vi "Facade 3.vi"(0 "Data In":T4, 2 "Display State In":T2, 3 "Container State":T3) -> (6 "Data Out":T4, 7 "Display State Out":T2, 8 "Action":T1)   [LabVIEW 2021, in "溫度計.xctl"]
uses:
  Data 3.ctl
  <vilib>/_xctls/Container State.ctl
  State 3.ctl
  <vilib>/_xctls/Action.ctl
  <vilib>/_xctls/XControlSupport.lvlib
panel:
  in  "下限":dbl
  in  "圖片異常":path
  in  "圖片正常":path
  out "訊息":string
  in  "上限":dbl
  out "顯示圖片":picture
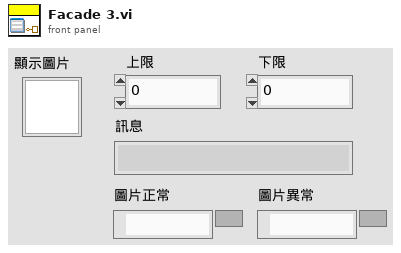
[diagram p1: front panel]
types:
  T1 = typedef "XControlSupport.lvlib/Action.ctl" = cluster{"Data Changed?":bool, "State Changed?":bool, "Action Name":string}
  T2 = typedef "溫度計.xctl/State 3.ctl" = cluster{"Numeric":dbl}
  T3 = typedef "XControlSupport.lvlib/Container State.ctl" = cluster{"Indicator?":bool, "Run Mode?":bool, " Refnum":refnum<vi>}
  T4 = typedef "溫度計.xctl/Data 3.ctl" = dbl
  T5 = typedef "imagedata.ctl" = cluster{"image type":i32, "image depth":i32, "image":u8[], "mask":u8[], "colors":u32[], "Rectangle":cluster{"left":i16, "top":i16, "right":i16, "bottom":i16}}
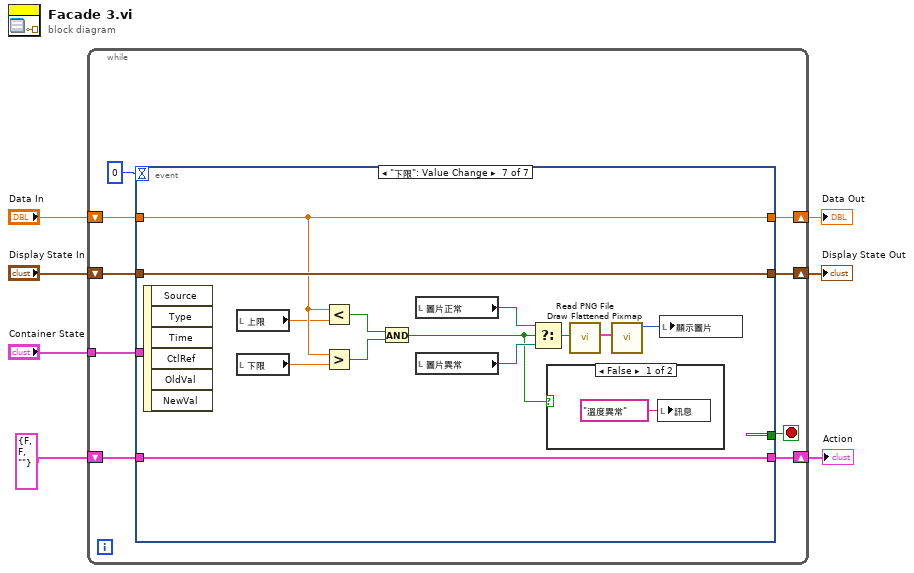
[diagram p0: block diagram]
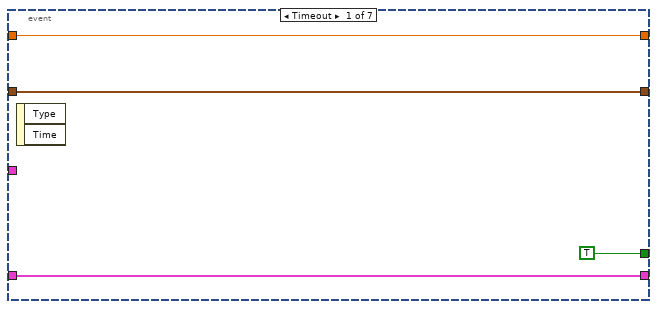
[diagram p2: hidden frame]
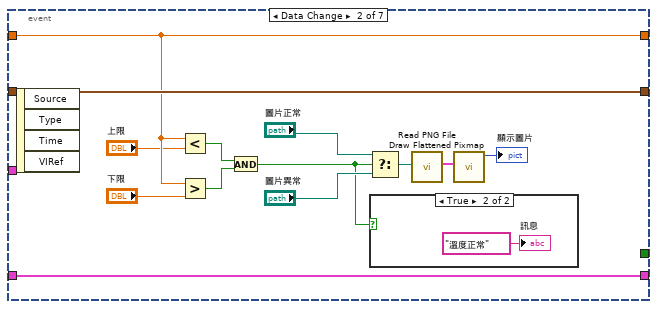
[diagram p3: hidden frame]
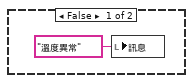
[diagram p4: hidden frame]
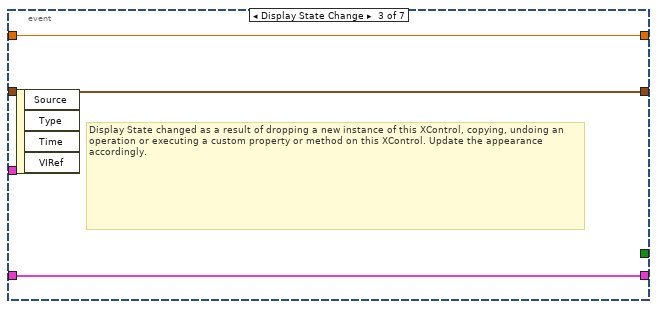
[diagram p5: hidden frame]
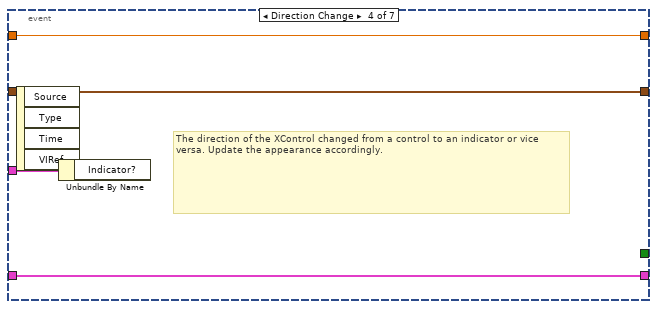
[diagram p6: hidden frame]
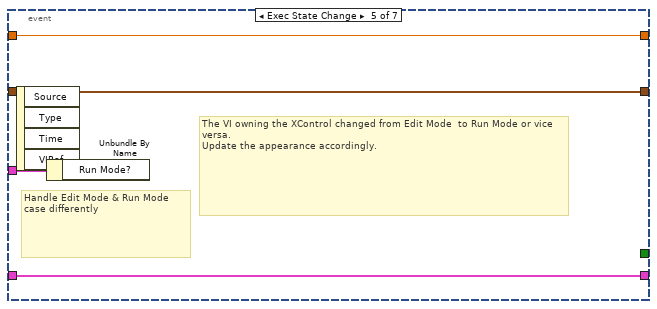
[diagram p7: hidden frame]
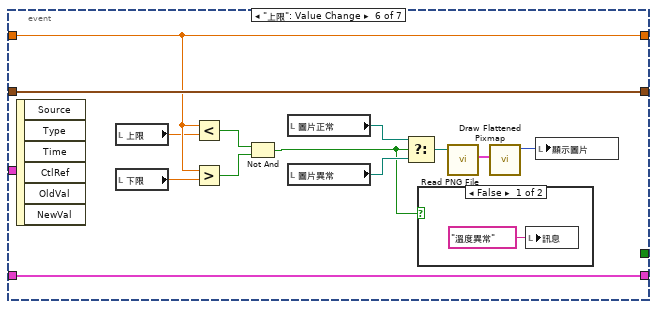
[diagram p8: hidden frame]
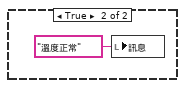
[diagram p9: hidden frame]
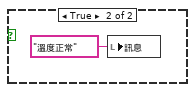
[diagram p10: hidden frame]
diagram:
  n1 = while {
    shift-right: [w15] -> w4
    shift-left: "Display State In" -> [w16]
    tunnel: "Container State" -> [w12]
    shift-right: [w10] -> w7
    shift-left: "Data In" -> [w11]
    shift-right: [w8] -> w2
    shift-left: T1 {"Data Changed?"=FALSE, "State Changed?"=FALSE, "Action Name"=""} ("Action") -> [w9]
    stop <- w14 stop-if-true
    n2 = event shown="[6] \"下限\": Value Change" {
      selector: _ -> [_ _ _ _ _ _ _]
      dyn-events: _ -> [_ _ _ _ _ _ _]
      timeout: 0 -> [_ _ _ _ _ _ _]
      tunnel: w16 -> [w18 w33 w38 w41 w45 w59 w74]
      tunnel: [w18 w33 w38 w41 w45 w59 w74] -> w15
      tunnel: [TRUE _ _ _ _ _ _] -> w14
      tunnel: w12 -> [_ _ _ w42 w46 _ _]
      tunnel: w11 -> [w17 w26 w37 w40 w44 w52 w67]
      tunnel: [w17 w26 w37 w40 w44 w52 w67] -> w10
      tunnel: [w19 w32 w36 w39 w43 w58 w73] -> w8
      tunnel: w9 -> [w19 w32 w36 w39 w43 w58 w73]
      event Timeout {
        n3 = event-data() -> ()  [unwired: 1 in, 2 out]
      }
      event Data Change {
        n4 = event-data() -> ()  [unwired: 1 in, 4 out]
        n5 = Less?(x=w26, y="上限") -> (x < y?=w23:bool)
        n6 = Greater?(x=w26, y="下限") -> (0:w22:bool)
        n7 = And(x=w23, y=w22) -> (x .and. y?=w21:bool)
        n8 = Select(t="圖片正常", s=w21, f="圖片異常") -> (s? t:f=w30:path)
        n9 = case shown="True" w21 {
          frame False {
            n10 = local write "訊息"("溫度異常" ("訊息")) -> ()
          }
          frame True {
            "訊息" <- "溫度正常" ("訊息")
          }
        }
        n11 = call <vilib>:"Read PNG File.vi"("path to PNG file"=w30) -> ("image data"=w27:T5)  [unwired: 8 in, 2 out]
        n12 = call <vilib>:"Draw Flattened Pixmap.vi"("image data"=w27) -> ("new picture"=→"顯示圖片":picture)  [unwired: 8 in]
      }
      event Display State Change {
        # "Display State changed as a result of dropping a new instance of this XControl, copying, undoing an operation or executing a custom property or method on this XControl. Update the appearance accordingly."
        n13 = event-data() -> ()  [unwired: 1 in, 4 out]
      }
      event Direction Change {
        # "The direction of the XControl changed from a control to an indicator or vice versa. Update the appearance accordingly."
        n14 = event-data() -> ()  [unwired: 1 in, 4 out]
        n15 = Unbundle By Name(w42) -> ()  [unwired: 1 out]
      }
      event Exec State Change {
        # "The VI owning the XControl changed from Edit Mode  to Run Mode or vice versa.\nUpdate the appearance accordingly."
        # "Handle Edit Mode & Run Mode\ncase differently"
        n16 = event-data() -> ()  [unwired: 1 in, 4 out]
        n17 = Unbundle By Name(w46) -> ()  [unwired: 1 out]
      }
      event "上限": Value Change {
        n18 = event-data() -> ()  [unwired: 1 in, 6 out]
        n19 = local read "上限"() -> (w51:dbl)
        n20 = local read "下限"() -> (w50:dbl)
        n21 = Less?(x=w52, y=w51) -> (x < y?=w49:bool)
        n22 = Greater?(x=w52, y=w50) -> (0:w48:bool)
        n23 = Not And(1:w48, 2:w49) -> (0:w47:bool)
        n24 = local read "圖片正常"() -> (w54:path)
        n25 = local read "圖片異常"() -> (w53:path)
        n26 = Select(t=w54, s=w47, f=w53) -> (s? t:f=w55:path)
        n27 = case shown="False" w47 {
          frame False {
            n28 = local write "訊息"("溫度異常" ("訊息")) -> ()
          }
          frame True {
            n29 = local write "訊息"("溫度正常" ("訊息")) -> ()
          }
        }
        n30 = call <vilib>:"Read PNG File.vi"("path to PNG file"=w55) -> ("image data"=w57:T5)  [unwired: 8 in, 2 out]
        n31 = call <vilib>:"Draw Flattened Pixmap.vi"("image data"=w57) -> ("new picture"=w56:picture)  [unwired: 8 in]
        n32 = local write "顯示圖片"(w56) -> ()
      }
      event "下限": Value Change {
        n33 = event-data() -> ()  [unwired: 1 in, 6 out]
        n34 = local read "上限"() -> (w66:dbl)
        n35 = local read "下限"() -> (w65:dbl)
        n36 = Less?(x=w67, y=w66) -> (x < y?=w64:bool)
        n37 = Greater?(x=w67, y=w65) -> (0:w63:bool)
        n38 = And(x=w64, y=w63) -> (x .and. y?=w62:bool)
        n39 = local read "圖片正常"() -> (w69:path)
        n40 = local read "圖片異常"() -> (w68:path)
        n41 = Select(t=w69, s=w62, f=w68) -> (s? t:f=w72:path)
        n42 = case shown="False" w62 {
          frame False {
            n43 = local write "訊息"("溫度異常" ("訊息")) -> ()
          }
          frame True {
            n44 = local write "訊息"("溫度正常" ("訊息")) -> ()
          }
        }
        n45 = call <vilib>:"Read PNG File.vi"("path to PNG file"=w72) -> ("image data"=w71:T5)  [unwired: 8 in, 2 out]
        n46 = call <vilib>:"Draw Flattened Pixmap.vi"("image data"=w71) -> ("new picture"=w70:picture)  [unwired: 8 in]
        n47 = local write "顯示圖片"(w70) -> ()
      }
    }
  }
  "Display State Out" <- w4
  "Data Out" <- w7
  "Action" <- w2
